vi "create_arb_waveform.vi"(0 "Waveform Parameters":T1={"Functional Form"=enum."Exponential", "Start Voltage"=0.0, "End Voltage"=0.0, "Time (s)"=0.0, "Degree (polynomial only)"=1, "Sample Rate"=0.0} {"Degree (polynomial only)" min=1}) -> (1 "Samples to Write":dbl, 2 "dt":dbl, 3 "Tau (exponential)":dbl, 4 "output waveform":waveform(dbl)(graph))   [LabVIEW 2013]
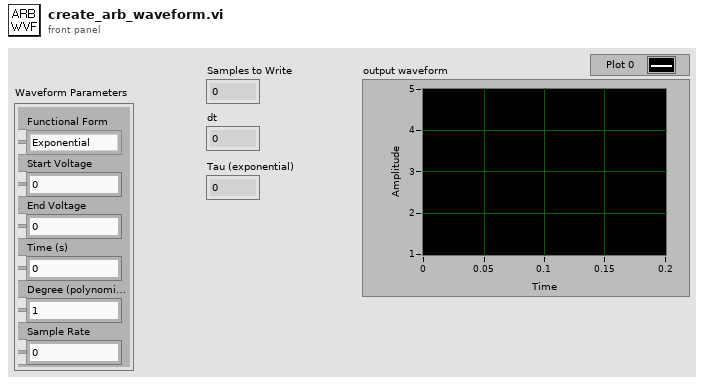
[diagram p1: front panel]
types:
  T1 = cluster{"Functional Form":enum16{"Polynomial", "Exponential"}, "Start Voltage":dbl, "End Voltage":dbl, "Time (s)":dbl, "Degree (polynomial only)":i8, "Sample Rate":dbl}
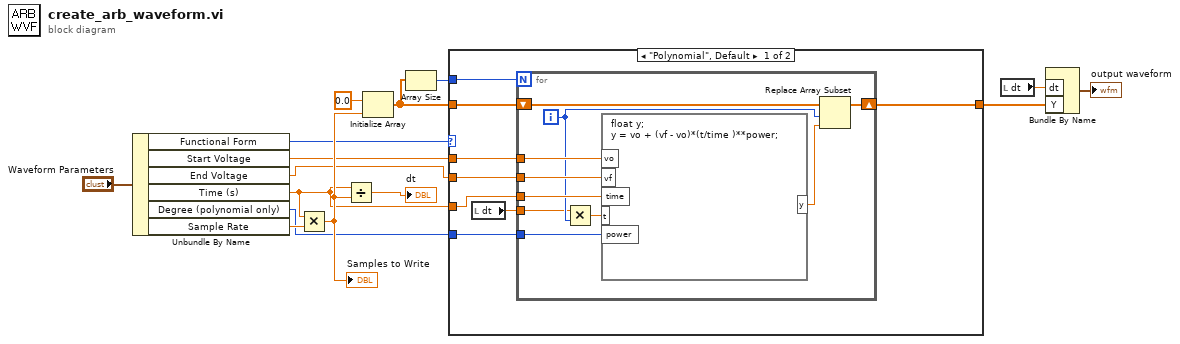
[diagram p0: block diagram]
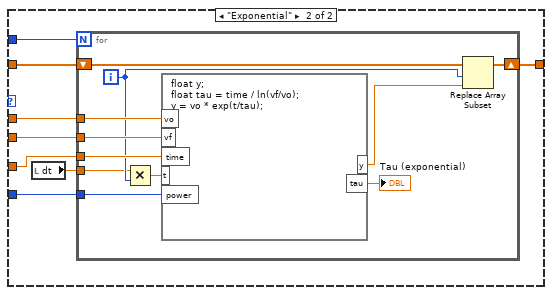
[diagram p2: hidden frame]
diagram:
  n1 = Unbundle By Name("Waveform Parameters") -> ("Functional Form"=w6:enum16{"Polynomial", "Exponential"}, "Start Voltage"=w1:dbl, "End Voltage"=w2:dbl, "Time (s)"=w5:dbl, "Degree (polynomial only)"=w3:i8, "Sample Rate"=w4:dbl)
  n2 = Multiply(x=w5, y=w4) -> (x*y=w13:dbl)
  "Samples to Write" <- w13
  n3 = Divide(x=w5, y=w13) -> (x/y=→"dt":dbl)
  n4 = Initialize Array(0.0 ("element"), w13) -> (w9:dbl[])
  n5 = Array Size(array=w9) -> (size(s)=w8:i32)
  n6 = case shown="\"Polynomial\", Default" w6 {
    tunnel: w9 -> [w23 w41]
    tunnel: [w22 w40] -> w14
    tunnel: w1 -> [w21 w39]
    tunnel: w2 -> [w20 w38]
    tunnel: w5 -> [w19 w37]
    tunnel: w3 -> [w17 w35]
    tunnel: w8 -> [w16 w34]
    frame "Polynomial", Default {
      n7 = local read "dt"() -> (w18:dbl)
      n8 = for {
        N: w16 -> [_]
        shift-right: [w32] -> w22
        shift-left: w23 -> [w33]
        tunnel: w21 -> [w31]
        tunnel: w20 -> [w30]
        tunnel: w19 -> [w29]
        tunnel: w18 -> [w26]
        tunnel: w17 -> [w25]
        i -> [w27]
        n9 = Multiply(x=w26, y=w27) -> (x*y=w28:dbl)
        n10 = formula code="float y;\ny = vo + (vf - vo)*(t/time )**power;"("vo"=w31, "vf"=w30, "time"=w29, "t"=w28, "power"=w25) -> ("y"=w24:dbl)
        n11 = Replace Array Subset(array=w33, new element=w24, index=w27) -> (w32:dbl[])
      }
    }
    frame "Exponential" {
      n12 = local read "dt"() -> (w36:dbl)
      n13 = for {
        N: w34 -> [_]
        shift-right: [w51] -> w40
        shift-left: w41 -> [w52]
        tunnel: w39 -> [w50]
        tunnel: w38 -> [w49]
        tunnel: w37 -> [w48]
        tunnel: w36 -> [w45]
        tunnel: w35 -> [w44]
        i -> [w46]
        n14 = Multiply(x=w45, y=w46) -> (x*y=w47:dbl)
        n15 = formula code="float y;\nfloat tau = time / ln(vf/vo);\ny = vo * exp(t/tau);"("vo"=w50, "vf"=w49, "time"=w48, "t"=w47, "power"=w44) -> ("y"=w43:dbl, "tau"=→"Tau (exponential)":dbl)
        n16 = Replace Array Subset(array=w52, new element=w43, index=w46) -> (w51:dbl[])
      }
    }
  }
  n17 = local read "dt"() -> (w11:dbl)
  n18 = Bundle By Name("dt"=w11, "Y"=w14) -> (→"output waveform":waveform(dbl))  [unwired: 1 in]
